vi "AVS_UpdateETHDevices.vi"(0 "ListSizeInput":u32, 7 "RequiredSizeInput":u32, 11 "ListInpit":u8[](array[numeric])) -> (4 "ListSizeOutput":u32, 8 "RequiredSizeOutput":u32, 15 "List Output":u8[](array[numeric]))   [LabVIEW 2016]
uses:
  libavs.so
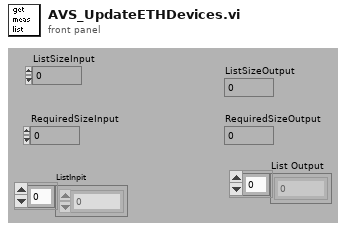
[diagram p1: front panel]
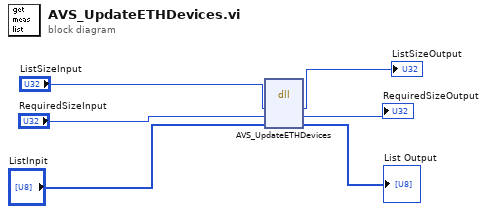
[diagram p0: block diagram]
diagram:
  n1 = dll-call lib="home/harini/tcs/ts_sedspectrometer/ss_sedspectrometer/VIs/libavs.so" fn="AVS_UpdateETHDevices"("a_ListSize"="ListSizeInput", "a_pRequiredSize"="RequiredSizeInput", "a_pList"="ListInpit") -> ("a_ListSize"=→"ListSizeOutput":u32, "a_pRequiredSize"=→"RequiredSizeOutput":u32, "a_pList"=→"List Output":u8[])  [unwired: 4 in, 2 out]
